vi "Update Preview.vi"(8 "error in (no error)":errorcluster, 11 "Editor in":refnum<class "Editor.lvclass">) -> (0 "error out":errorcluster, 3 "Editor out":refnum<class "Editor.lvclass">)   [LabVIEW 2020, in "VolatusGUIEditor.lvlib" / "Editor.lvclass"]
uses:
  Editor.lvclass
  Editor.lvclass/Editor.ctl
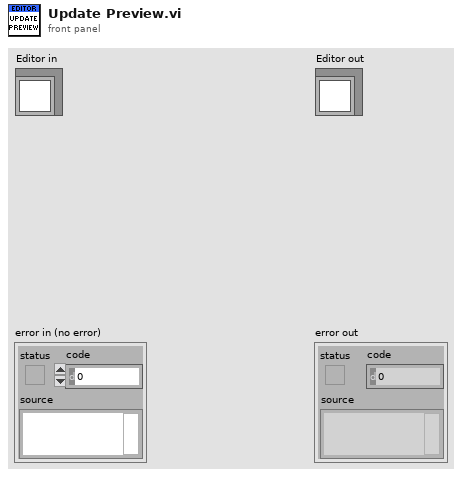
[diagram p1: front panel]
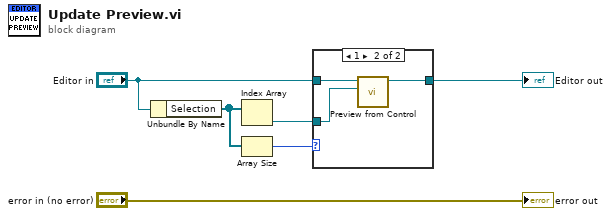
[diagram p0: block diagram]
diagram:
  n1 = Unbundle By Name("Editor in") -> ("Selection"=w3:refnum<vi>[])
  n2 = Index Array(array=w3) -> (element=w1:refnum<vi>)  [unwired: 1 in]
  n3 = Array Size(array=w3) -> (size(s)=w2:i32)
  n4 = case shown="1" w2 {
    tunnel: "Editor in" -> [w7 w10]
    tunnel: [w7 w9] -> w4
    tunnel: w1 -> [_ w8]
    frame Default {
    }
    frame 1 {
      n5 = call "Preview from Control.vi"("Ctl Refnum"=w8, "Editor in"=w10) -> ("Editor out"=w9:refnum<class "Editor.lvclass">)  [unwired: 8 in, 1 out]
    }
  }
  "Editor out" <- w4
  "error out" <- "error in (no error)"
